vi "Const_ADO.vi"() -> (0 "ADOMapper":refnum<class "ADOMapper.lvclass">)   [LabVIEW 2020, in "ORM_ADONet.lvlib"]
uses:
  ADOMapper/ADOMapper.lvclass
  ORM_ADONet.lvlib
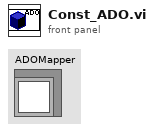
[diagram p1: front panel]
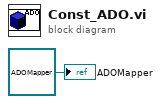
[diagram p0: block diagram]
diagram:
  "ADOMapper" <- refnum<class "ADOMapper.lvclass"> refnum ("ADONet.lvlib:ADOMapper.lvclass")
